vi "Init.vi"(8 "error in (no error)":errorcluster, 10 "ID":string, 11 "Effect Unit in":refnum<class "Effect Unit.lvclass">) -> (0 "error out":errorcluster, 3 "Effect Unit out":refnum<class "Effect Unit.lvclass">)   [LabVIEW 2020, in "Effect Unit.lvclass"]
uses:
  Effect Unit.lvclass
  Effect Info.ctl
  Packed Libraries/Messaging.lvlibp/Message Cluster.ctl
  Plugin Interfaces/Effect Interface/Effect Interface.lvlibp/Effect Interface Class/Effect Interface.lvclass
  Effect Unit.lvclass/Effect Unit.ctl
  Packed Libraries/Messaging.lvlibp
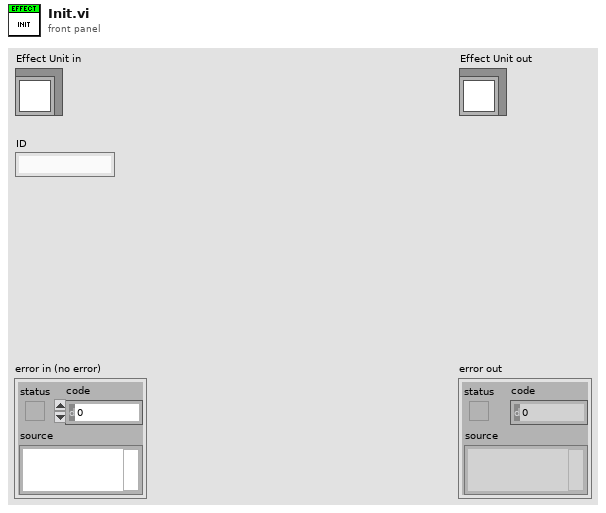
[diagram p1: front panel]
types:
  T1 = typedef "Effect Unit.lvclass/Effect Info.ctl" = cluster{"ID":string, "Message Queue":refnum<queue>, "Effect Interface":refnum<class "Effect Interface.lvclass">}
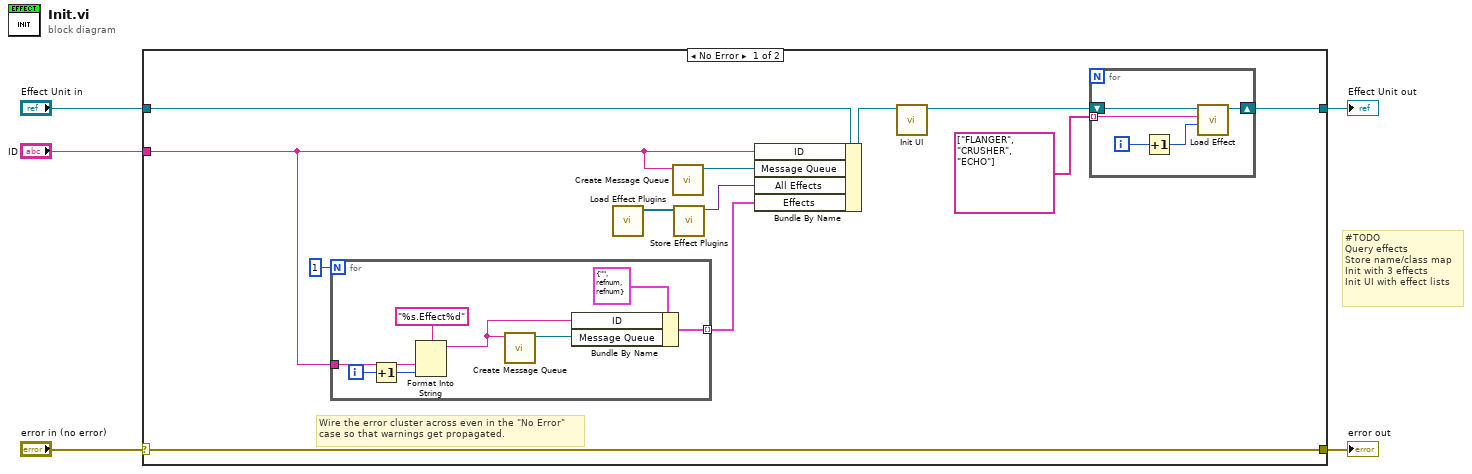
[diagram p0: block diagram]
diagram:
  # "#TODO\nQuery effects\nStore name/class map\nInit with 3 effects\nInit UI with effect lists"
  n1 = case shown="No Error" "error in (no error)" {
    selector: "error in (no error)" -> [w17 w32]
    tunnel: [w17 w32] -> w4
    tunnel: [w9 w31] -> w2
    tunnel: "Effect Unit in" -> [w15 w31]
    tunnel: "ID" -> [w14 _]
    frame No Error {
      # "Wire the error cluster across even in the \"No Error\"\ncase so that warnings get propagated."
      n2 = for {
        N: 1 -> [_]
        tunnel: w14 -> [w29]
        tunnel: [w23] -> w12 mode=indexing
        i -> [w28]
        n3 = Increment(x=w28) -> (x+1=w27:i32)
        n4 = Format Into String(format string="%s.Effect%d", w29, w27) -> (resulting string=w25:string)  [unwired: 2 in, 1 out]
        n5 = call "Create Message Queue.vi"("Queue Name"=w25) -> ("queue out"=w26:refnum<queue>)  [unwired: 9 in, 1 out]
        n6 = Bundle By Name(cluster=T1 {"ID"="", "Message Queue"=refnum, "Effect Interface"=refnum} ("Effect Info"), "ID"=w25, "Message Queue"=w26) -> (w23:T1)
      }
      n7 = call "Load Effect Plugins.vi"() -> ("Effect Plugins"=w13:refnum<class "Effect Interface.lvclass">[])  [unwired: 11 in]
      n8 = call "Create Message Queue.vi"("Queue Name"=w14) -> ("queue out"=w16:refnum<queue>)  [unwired: 9 in, 1 out]
      n9 = call "Store Effect Plugins.vi"("Effects"=w13) -> ("Effect Plugin Map"=w11:variant)  [unwired: 10 in]
      n10 = Bundle By Name(cluster=w15, "ID"=w14, "Message Queue"=w16, "All Effects"=w11, "Effects"=w12) -> (w7:refnum<class "Effect Unit.lvclass">)
      n11 = call "Init UI.vi"("Effect Unit in"=w7) -> ("Effect Unit out"=w6:refnum<class "Effect Unit.lvclass">)  [unwired: 9 in, 1 out]
      n12 = for {
        tunnel: string[] ["FLANGER", "CRUSHER", "ECHO"] -> [w20] mode=indexing
        shift-right: [w21] -> w9
        shift-left: w6 -> [w22]
        i -> [w19]
        n13 = Increment(x=w19) -> (x+1=w18:i32)
        n14 = call "Load Effect.vi"("Effect Slot"=w18, "Effect Name"=w20, "Effect Unit in"=w22) -> ("Effect Unit out"=w21:refnum<class "Effect Unit.lvclass">)  [unwired: 7 in, 1 out]
      }
    }
    frame Error {
    }
  }
  "error out" <- w4
  "Effect Unit out" <- w2
